vi "SetMoveSettings.vi"(7 "Mode":T1, 8 "error in (no error)":errorcluster, 9 "Calibration":cluster{dbl, "MicrostepMode":u32}[](array[cluster]), 10 "Speed":sgl, 11 "IDs":i32[](array[numeric])) -> (0 "error out":errorcluster, 2 "Move Settings":T2(array[cluster]), 3 "Success?":bool)   [LabVIEW 2020]
uses:
  SettingCtrlOptions.ctl
  libximc.lvlib
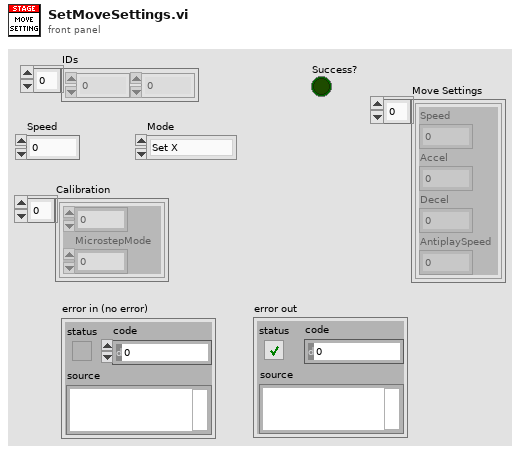
[diagram p1: front panel]
types:
  T1 = typedef "SettingCtrlOptions.ctl" = enum16{"Set X", "Set Y", "Set X and Y", "Get Settings", "None"}
  T2 = cluster{"Speed":sgl, "Accel":sgl, "Decel":sgl, "AntiplaySpeed":sgl}[]
  T3 = cluster{"Speed":sgl, "Accel":sgl, "Decel":sgl, "AntiplaySpeed":sgl}
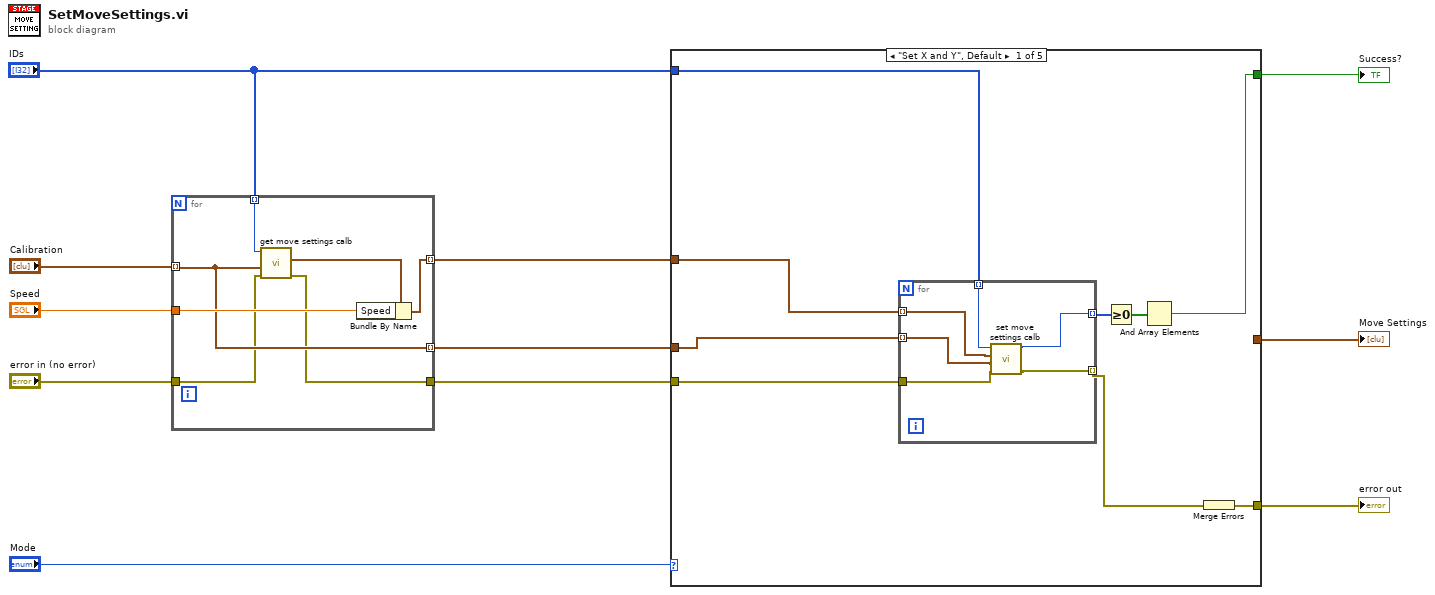
[diagram p0: block diagram]
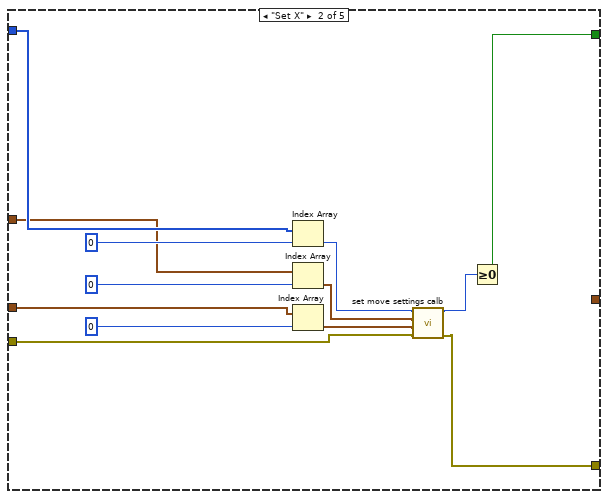
[diagram p2: hidden frame]
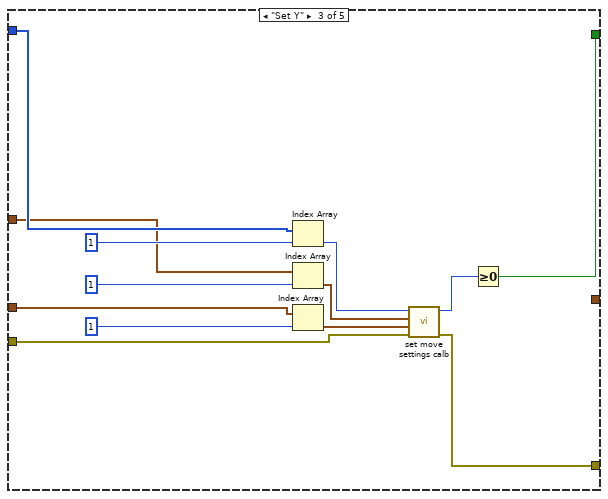
[diagram p3: hidden frame]
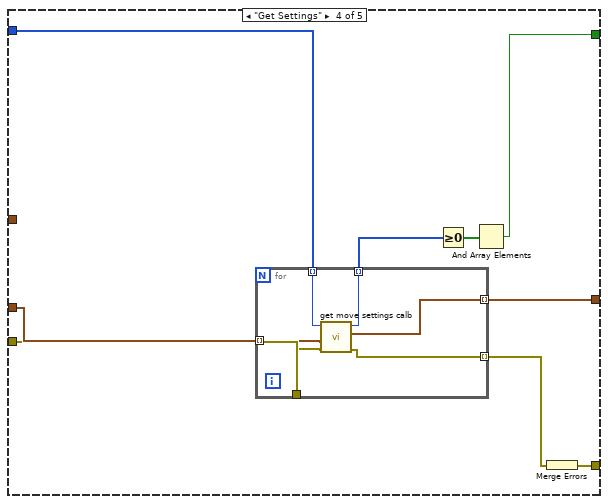
[diagram p4: hidden frame]
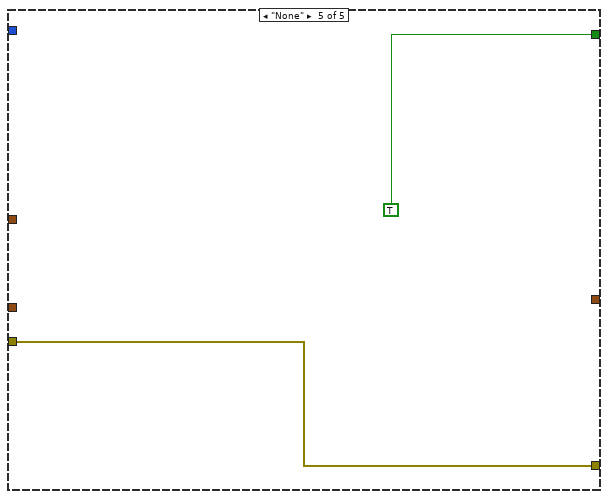
[diagram p5: hidden frame]
diagram:
  n1 = for {
    tunnel: [w17] -> w6 mode=indexing
    tunnel: "IDs" -> [w18] mode=indexing
    tunnel: "Speed" -> [w15]
    tunnel: "Calibration" -> [w14] mode=indexing
    tunnel: [w14] -> w3 mode=indexing
    tunnel: "error in (no error)" -> [w13]
    tunnel: [w12] -> w1
    n2 = call "get move settings calb.vi"("error in (no error)"=w13, "calibration"=w14, "id"=w18) -> ("error out"=w12:errorcluster, "move_settings_calb out"=w16:T3)  [unwired: 6 in, 1 out]
    n3 = Bundle By Name(cluster=w16, "Speed"=w15) -> (w17:T3)
  }
  n4 = case shown="\"Set X and Y\", Default" "Mode" {
    tunnel: w6 -> [w27 w43 w56 _ _]
    tunnel: "IDs" -> [w26 w46 w59 w65 _]
    tunnel: w1 -> [w25 w38 w52 w63 w76]
    tunnel: [w22 w34 w51 w62 w76] -> w11
    tunnel: w3 -> [w23 w41 w54 w64 _]
    tunnel: [w19 w40 w53 w67 TRUE] -> w10
    tunnel: [_ _ _ w60 _] -> w9
    frame "Set X and Y", Default {
      n5 = for {
        tunnel: w27 -> [w30] mode=indexing
        tunnel: [w33] -> w24 mode=indexing
        tunnel: w26 -> [w29] mode=indexing
        tunnel: w25 -> [w32]
        tunnel: [w28] -> w20 mode=indexing
        tunnel: w23 -> [w31] mode=indexing
        n6 = call "set move settings calb.vi"("error in (no error)"=w32, "calibration"=w31, "move_settings_calb"=w30, "id"=w29) -> ("error out"=w33:errorcluster, "function return"=w28:i32)  [unwired: 6 in]
      }
      n7 = Greater Or Equal To 0?(x=w20) -> (x >= 0?=w21:bool[])
      n8 = And Array Elements(Boolean array=w21) -> (logical AND=w19:bool)
      n9 = Merge Errors(w24) -> (w22:errorcluster)
    }
    frame "Set X" {
      n10 = Index Array(array=w46, index=0) -> (element=w39:i32)
      n11 = Index Array(array=w43, index=0) -> (element=w36:T3)
      n12 = Index Array(array=w41, index=0) -> (element=w37:cluster{dbl, "MicrostepMode":u32})
      n13 = call "set move settings calb.vi"("error in (no error)"=w38, "calibration"=w37, "move_settings_calb"=w36, "id"=w39) -> ("error out"=w34:errorcluster, "function return"=w35:i32)  [unwired: 6 in]
      n14 = Greater Or Equal To 0?(x=w35) -> (x >= 0?=w40:bool)
    }
    frame "Set Y" {
      n15 = Index Array(array=w59, index=1) -> (element=w50:i32)
      n16 = Index Array(array=w56, index=1) -> (element=w48:T3)
      n17 = Index Array(array=w54, index=1) -> (element=w49:cluster{dbl, "MicrostepMode":u32})
      n18 = call "set move settings calb.vi"("error in (no error)"=w52, "calibration"=w49, "move_settings_calb"=w48, "id"=w50) -> ("error out"=w51:errorcluster, "function return"=w47:i32)  [unwired: 6 in]
      n19 = Greater Or Equal To 0?(x=w47) -> (x >= 0?=w53:bool)
    }
    frame "Get Settings" {
      n20 = for {
        tunnel: w65 -> [w71] mode=indexing
        tunnel: [w73] -> w61 mode=indexing
        tunnel: w63 -> [w74]
        tunnel: w64 -> [w72] mode=indexing
        tunnel: [w69] -> w60 mode=indexing
        tunnel: [w70] -> w66 mode=indexing
        n21 = call "get move settings calb.vi"("error in (no error)"=w74, "calibration"=w72, "id"=w71) -> ("error out"=w73:errorcluster, "move_settings_calb out"=w69:T3, "function return"=w70:i32)  [unwired: 6 in]
      }
      n22 = Greater Or Equal To 0?(x=w66) -> (x >= 0?=w68:bool[])
      n23 = And Array Elements(Boolean array=w68) -> (logical AND=w67:bool)
      n24 = Merge Errors(w61) -> (w62:errorcluster)
    }
    frame "None" {
    }
  }
  "error out" <- w11
  "Success?" <- w10
  "Move Settings" <- w9
